vi "Plot menu selection.vi"(5 "Location":T1, 7 "VI ref":refnum<vi>, 8 "error in (no error)":errorcluster, 9 "ItemPath":string, 10 "ItemTag":string, 11 "StokePlotHandle in":refnum<class "BjusticePlotHandle.lvclass">) -> (0 "error out":errorcluster, 3 "StokePlotHandle out":refnum<class "BjusticePlotHandle.lvclass">)   [LabVIEW 2021, in "BjusticePlotHandle.lvclass"]
uses:
  BjusticePlotHandle.lvclass
  TypeDefs/Shortcut Location.ctl
  SubVIs/menu/Plot menu activation submenu type v2.ctl
  TypeDefs/Plot axis.ctl
  1PLOT to MPLOT UE.ctl
  1PLOT to MPLOT type.ctl
  BjusticePlotHandle.lvclass/BjusticePlotHandle.ctl
  RocketPlot.lvlib
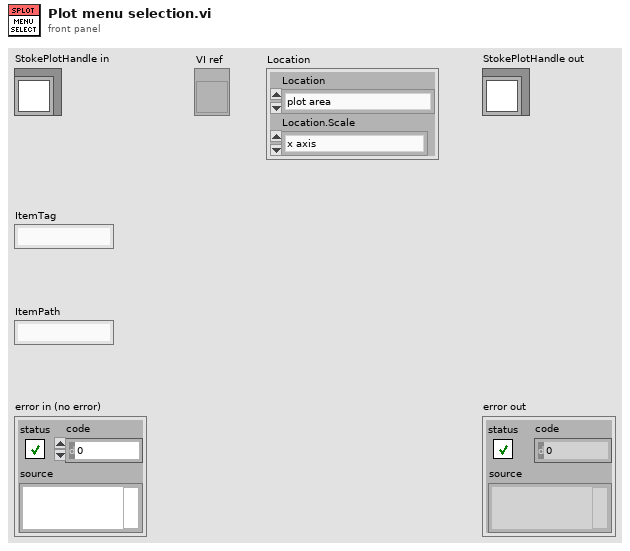
[diagram p1: front panel]
types:
  T1 = typedef "RocketPlot.lvlib/Shortcut Location.ctl" = cluster{"Location":T2, "Location.Scale":T3}
  T2 = typedef "RocketPlot.lvlib/Plot menu activation submenu type v2.ctl" = enum16{"plot area", "plot border", "markers", "scale"}
  T3 = typedef "RocketPlot.lvlib/Plot axis.ctl" = enum16{"x axis", "left axis", "right axis"}
  T4 = typedef "BjusticePlotHandle.lvclass/1PLOT to MPLOT type.ctl" = enum16{"Maximize", "ShortcutMenu"}
  T5 = typedef "BjusticePlotHandle.lvclass/1PLOT to MPLOT UE.ctl" = cluster{"Type":T4, "source VI ref":refnum<vi>, "data":variant}
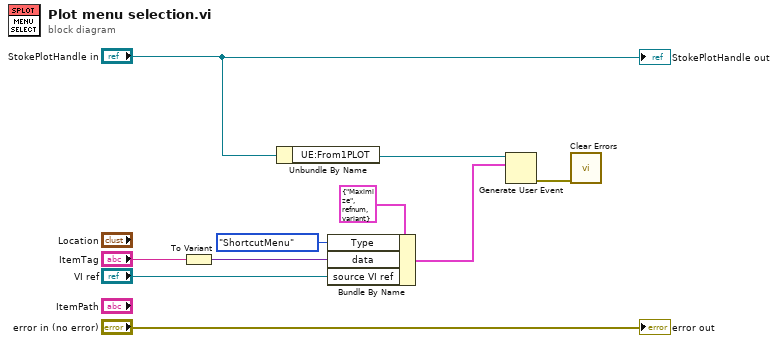
[diagram p0: block diagram]
diagram:
  n1 = To Variant(anything="ItemTag") -> (Variant=w2:variant)
  n2 = Unbundle By Name("StokePlotHandle in") -> ("UE:From1PLOT"=w10:refnum<user-event>)
  n3 = Bundle By Name(cluster=T5 {"Type"=enum."Maximize", "source VI ref"=refnum, "data"=variant(string "")} ("event data"), "Type"=1PLOT_to_MPLOT_type."ShortcutMenu", "data"=w2, "source VI ref"="VI ref") -> (w4:T5)
  n4 = Generate User Event(user event=w10, event data cluster=w4) -> (error out=w8:errorcluster)  [unwired: 2 in, 1 out]
  n5 = call <vilib>:"Clear Errors.vi"("error in (no error)"=w8) -> ()  [unwired: 5 in, 2 out]
  "error out" <- "error in (no error)"
  "StokePlotHandle out" <- "StokePlotHandle in"
